vi "Controller panel.vi"() -> ()   [LabVIEW 2018]
uses:
  States.ctl
panel:
  out "Police reacting":bool
  out "Repairing":bool
  out "Traffic light failure":bool
  out "Accident":bool
  in  "Showsettings":bool
  in  "Logout":bool
  out "Current state":T1=enum."Night"
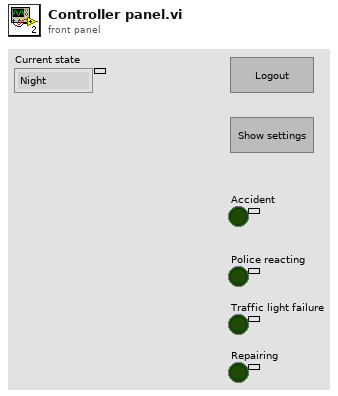
[diagram p1: front panel]
types:
  T1 = typedef "States.ctl" = enum16{"Normal", "Night", "Traffic jam 1", "Traffic jam 2"}
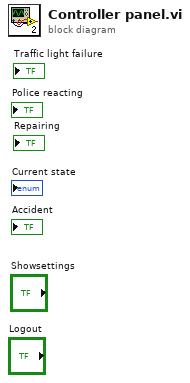
[diagram p0: block diagram]
diagram:
